vi "FGV-GEvt Refs(lvlibp).vi"(8 "error in (no error)":errorcluster) -> (0 "error out":errorcluster, 3 "CSM Global Log Ref":T1)   [LabVIEW 2017, in "Communicable State Machine.lvlib"]
doc: "-- <b>Controls</b> --\n- <b>Create(F)</b>:\n\n-- <b>Indicators</b> --\n- <b>CSM Global Log Event</b>:"
uses:
  Communicable State Machine.lvlib
  GEvt-Refs.ctl
  Typedef/_CSM_GlobalLog_MSG.ctl
  Typedef/_CSM_Response Source Message.ctl
  Typedef/_CSM_GlobalLog_MSG_TYPE.ctl
  FGV-GEvt Refs.vi
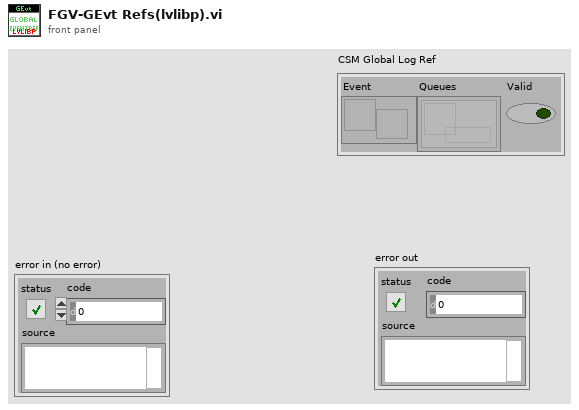
[diagram p1: front panel]
types:
  T1 = typedef "Communicable State Machine.lvlib/GEvt-Refs.ctl" = cluster{"Event":refnum<user-event>, "Queues":refnum<queue>[], "Valid":bool}
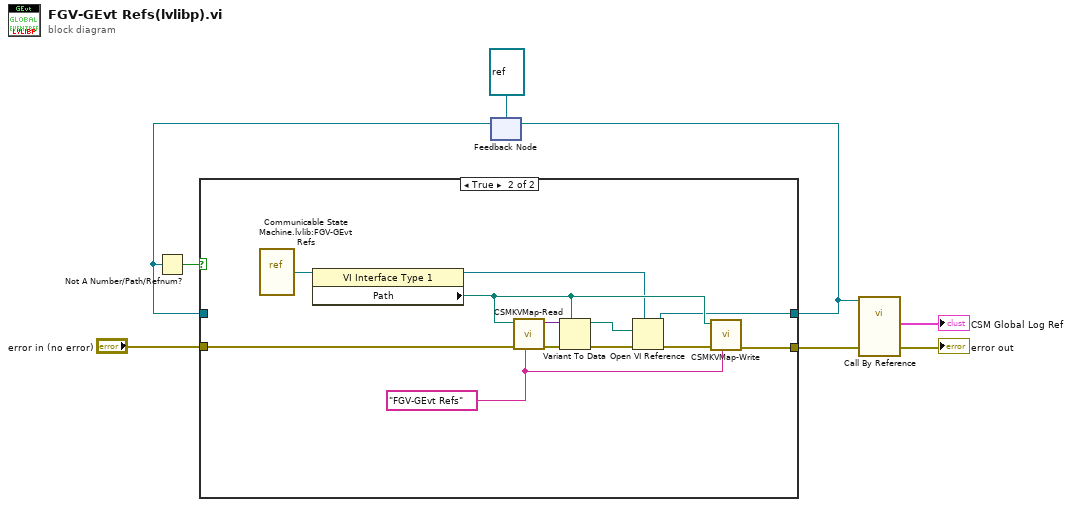
[diagram p0: block diagram]
diagram:
  n1 = feedback #1(refnum<vi> refnum) -> (w5:refnum<vi>)
  n2 = Not A Number/Path/Refnum?(number/path/refnum=w5) -> (NaN/Path/Refnum?=w8:bool)
  n3 = case shown="True" w8 {
    tunnel: [w9 w15] -> w4
    tunnel: [w10 w13] -> w3
    tunnel: "error in (no error)" -> [w10 w12]
    tunnel: w5 -> [w9 _]
    frame False {
    }
    frame True {
      w17 = "FGV-GEvt Refs" ("name")
      n4 = vi-ref "Communicable State Machine.lvlib:FGV-GEvt Refs.vi"() -> (w11:refnum<vi>)
      n5 = property class="VI Interface Type 1"(reference=w11) -> (reference out=w14:refnum<vi>, "Path"=w16:path)  [unwired: 1 in, 1 out]
      n6 = call "CSMKVMap-Read.vi"("name"=w17, "Error in"=w12, "default value (empty variant)"=w16) -> ("Error out"=w22:errorcluster, "value"=w21:variant)  [unwired: 5 in]
      n7 = Variant To Data(error in=w22, type=w16, Variant=w21) -> (data=w20:path, error out=w19:errorcluster)
      n8 = Open VI Reference(type specifier VI Refnum (for type only)=w14, vi path=w20, error in (no error)=w19) -> (vi reference=w15:refnum<vi>, error out=w18:errorcluster)  [unwired: 3 in]
      n9 = call "CSMKVMap-Write.vi"("name"=w17, "Error in"=w18, "value"=w16) -> ("Error out"=w13:errorcluster)  [unwired: 6 in]
    }
  }
  n10 = feedback-in #1(w4) -> ()
  n11 = call-by-ref "?"(reference=w4, "error in (no error)"=w3) -> ("error out"=→"error out":errorcluster, "CSM Global Log Ref"=→"CSM Global Log Ref":T1)  [unwired: 10 in, 2 out]
